vi "ViHandler.UnRegisterVi.Main.vi"(8 "ErrorIn":errorcluster, 10 "FinalExit?":bool=TRUE, 11 "ViInfo":T1) -> (0 "ErrorOut":errorcluster, 3 "UnregisterSuccessful?":bool)   [LabVIEW 2016, in "ViHandler.lvclass"]
uses:
  ViHandler.lvclass
  ViHandler.ViInfo.ctl
  ObjectHandler/ObjectHandler.GetObjectWType.ctl
  ObjectHandler/ObjectHandler.ObjectWType.ctl
  ObjectHandler/ObjectHandler.ObjectType.ctl
  ObjectHandler/ObjectHandler.lvclass
panel:
  out "ViHandlerRef":refnum<data-value>
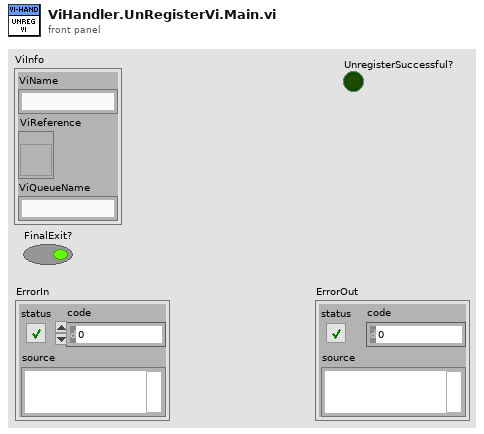
[diagram p1: front panel]
types:
  T1 = typedef "ViHandler.lvclass/ViHandler.ViInfo.ctl" = cluster{"ViName":string, "ViReference":refnum<vi>, "ViQueueName":string}
  T2 = typedef "ObjectHandler.lvclass/ObjectHandler.GetObjectWType.ctl" = cluster{"Name":string, "Caller":string}
  T3 = typedef "ObjectHandler.lvclass/ObjectHandler.ObjectWType.ctl" = cluster{"ObjectType":T4, "Object":variant}
  T4 = typedef "ObjectHandler.lvclass/ObjectHandler.ObjectType.ctl" = enum16{"undefined", "ObjectHandler", "ViHandler", "ErrorHandler", "CentralStorage", "Hausmodell", "Sondenmodell", "Wärmepumpe", "Umgebung"}
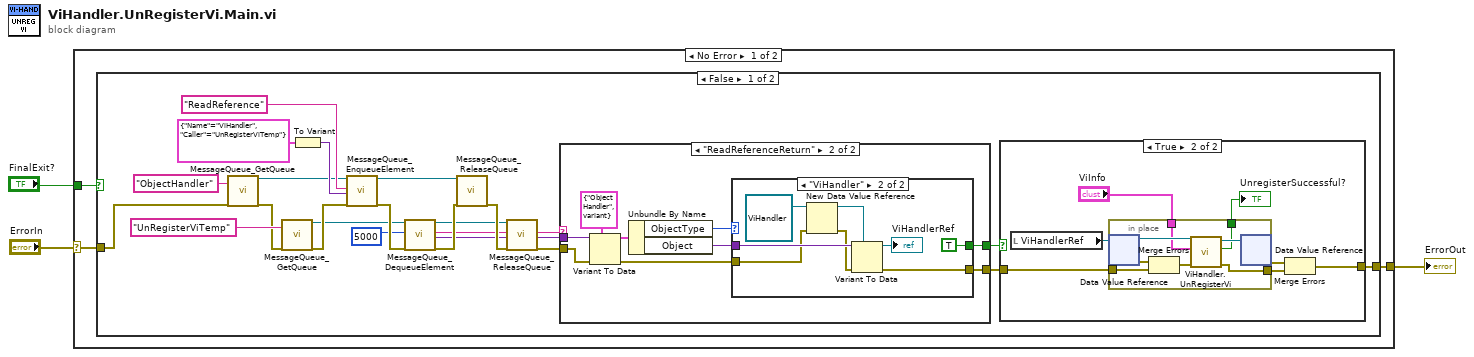
[diagram p0: block diagram]
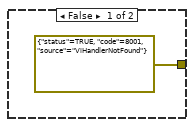
[diagram p2: hidden frame]
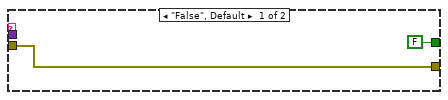
[diagram p3: hidden frame]
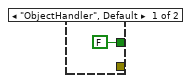
[diagram p4: hidden frame]
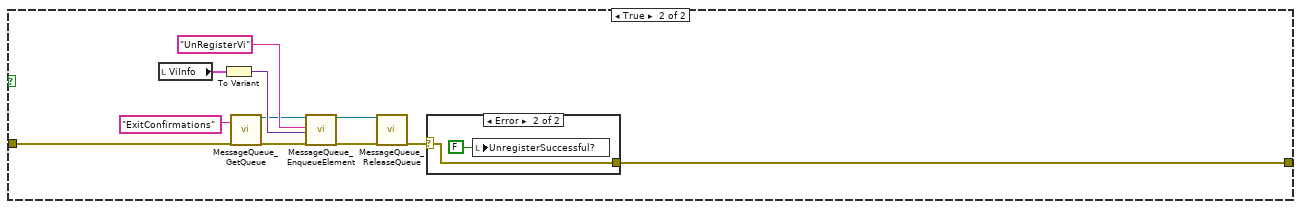
[diagram p5: hidden frame]
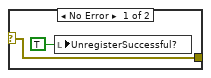
[diagram p6: hidden frame]
diagram:
  n1 = case shown="No Error" "ErrorIn" {
    selector: "ErrorIn" -> [w5 w80]
    tunnel: [w6 w80] -> w3
    tunnel: "FinalExit?" -> [w4 _]
    frame No Error {
      n2 = case shown="False" w4 {
        tunnel: [w8 w65] -> w6
        tunnel: w5 -> [w7 w73]
        frame False {
          n3 = call "MessageQueue_GetQueue.vi"("Name"="ObjectHandler", "ErrorIn"=w7) -> ("QueueOut"=w12:refnum<queue>, "ErrorOut"=w13:errorcluster)  [unwired: 15 in, 1 out]
          n4 = call "MessageQueue_GetQueue.vi"("Name"="UnRegisterViTemp" ("Caller"), "ErrorIn"=w13) -> ("QueueOut"=w18:refnum<queue>, "ErrorOut"=w22:errorcluster)  [unwired: 15 in, 1 out]
          n5 = To Variant(anything=T2 {"Name"="ViHandler", "Caller"="UnRegisterViTemp"} ("GetRefInput")) -> (Variant=w23:variant)
          n6 = call "MessageQueue_EnqueueElement.vi"("QueueIn"=w12, "Message"="ReadReference", "Data"=w23, "ErrorIn"=w22) -> ("QueueOut"=w15:refnum<queue>, "ErrorOut"=w20:errorcluster)  [unwired: 14 in]
          n7 = call "MessageQueue_DequeueElement.vi"("QueueIn"=w18, "Timeout"=5000, "ErrorIn"=w20) -> ("QueueOut"=w14:refnum<queue>, "Message"=w17:string, "Data"=w16:variant, "ErrorOut"=w28:errorcluster)  [unwired: 12 in, 1 out]
          n8 = call "MessageQueue_ReleaseQueue.vi"("QueueIn"=w15, "ErrorIn"=w28) -> ("ErrorOut"=w27:errorcluster)  [unwired: 15 in, 2 out]
          n9 = call "MessageQueue_ReleaseQueue.vi"("QueueIn"=w14, "ErrorIn"=w27) -> ("ErrorOut"=w11:errorcluster)  [unwired: 15 in, 2 out]
          n10 = case shown="\"ReadReferenceReturn\"" w17 {
            tunnel: w16 -> [_ w55]
            tunnel: [w45 w51] -> w10
            tunnel: w11 -> [w45 w49]
            tunnel: [FALSE w47] -> w9
            frame "False", Default {
            }
            frame "ReadReferenceReturn" {
              n11 = Variant To Data(error in=w49, type=T3 {"ObjectType"=enum."ObjectHandler", "Object"=variant} ("ObjectWType"), Variant=w55) -> (data=w54:T3, error out=w48:errorcluster)
              n12 = Unbundle By Name(w54) -> ("ObjectType"=w53:T4, "Object"=w52:variant)
              n13 = case shown="\"ViHandler\"" w53 {
                tunnel: w52 -> [_ w64]
                tunnel: [_ w61] -> w51
                tunnel: w48 -> [_ w60]
                tunnel: [FALSE TRUE] -> w47
                frame "ObjectHandler", Default {
                }
                frame "ViHandler" {
                  n14 = New Data Value Reference(data value=refnum<class "ViHandler.lvclass"> refnum ("ViHandler.lvclass"), error in=w60) -> (data value reference=w62:refnum<data-value>, error out=w59:errorcluster)
                  n15 = Variant To Data(error in=w59, type=w62, Variant=w64) -> (data=→"ViHandlerRef":refnum<data-value>, error out=w61:errorcluster)
                }
              }
            }
          }
          n16 = case shown="True" w9 {
            tunnel: w10 -> [_ w34]
            tunnel: [errorcluster {"status"=TRUE, "code"=8001, "source"="ViHandlerNotFound"} ("error IO") w32] -> w8
            frame False {
            }
            frame True {
              n17 = local read "ViHandlerRef"() -> (w33:refnum<data-value>)
              n18 = in-place {
                in-place-border: [w41] -> w36
                in-place-border: w34 -> [w43]
                in-place-border: "ViInfo" -> [w38]
                in-place-border: [w37] -> w30
                n19 = in-place-dvr #1(w33) -> (w39:refnum<class "ViHandler.lvclass">, w44:errorcluster)
                n20 = Merge Errors(w44, w43) -> (w42:errorcluster)
                n21 = call "ViHandler.UnRegisterVi.vi"("error in (no error)"=w42, "ViInfo"=w38, "ViHandler in"=w39) -> ("error out"=w41:errorcluster, "UnregisterSuccessful?"=w37:bool, "ViHandler out"=w40:refnum<class "ViHandler.lvclass">)  [unwired: 6 in]
                n22 = in-place-dvr #1(w40) -> (w35:errorcluster)  [unwired: 1 out]
              }
              "UnregisterSuccessful?" <- w30
              n23 = Merge Errors(w35, w36) -> (w32:errorcluster)
            }
          }
        }
        frame True {
          n24 = local read "ViInfo"() -> (w70:T1)
          n25 = To Variant(anything=w70) -> (Variant=w69:variant)
          n26 = call "MessageQueue_GetQueue.vi"("Name"="ExitConfirmations", "ErrorIn"=w73) -> ("QueueOut"=w68:refnum<queue>, "ErrorOut"=w72:errorcluster)  [unwired: 15 in, 1 out]
          n27 = call "MessageQueue_EnqueueElement.vi"("QueueIn"=w68, "Message"="UnRegisterVi", "Data"=w69, "ErrorIn"=w72) -> ("QueueOut"=w67:refnum<queue>, "ErrorOut"=w71:errorcluster)  [unwired: 14 in]
          n28 = call "MessageQueue_ReleaseQueue.vi"("QueueIn"=w67, "ErrorIn"=w71) -> ("ErrorOut"=w66:errorcluster)  [unwired: 15 in, 2 out]
          n29 = case shown="Error" w66 {
            selector: w66 -> [w76 w79]
            tunnel: [w76 w79] -> w65
            frame No Error {
              n30 = local write "UnregisterSuccessful?"(TRUE ("UnregisterSuccessful?")) -> ()
            }
            frame Error {
              n31 = local write "UnregisterSuccessful?"(FALSE ("UnregisterSuccessful?")) -> ()
            }
          }
        }
      }
    }
    frame Error {
    }
  }
  "ErrorOut" <- w3
